vi "Cleanup.vi"(8 "error in (no error)":errorcluster, 11 "Shadow in":refnum<class "Shadow.lvclass">) -> (0 "error out":errorcluster)   [LabVIEW 2021, in "UIShadow.lvlib" / "Shadow.lvclass"]
uses:
  Shadow.lvclass
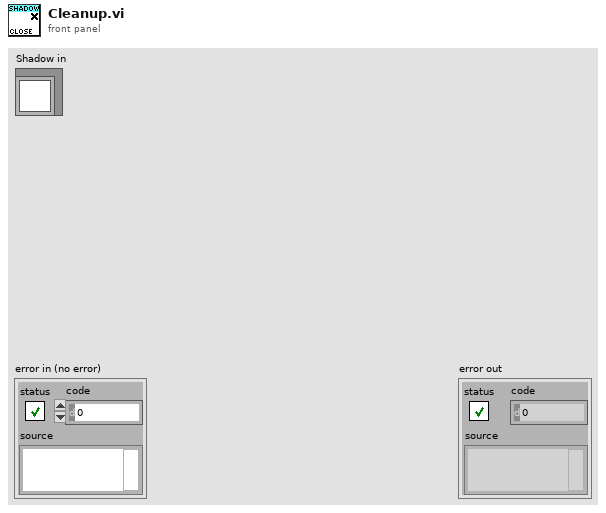
[diagram p1: front panel]
types:
  T1 = typedef "UIShadow.lvlib/Shadow.lvclass/Data.ctl" = cluster{"VI Refnum":refnum<vi>, "ShadowColor":u32, "Offset":i16, "Transparancy":i32, "UIShadowRef":refnum<vi>, "Activate?":bool}
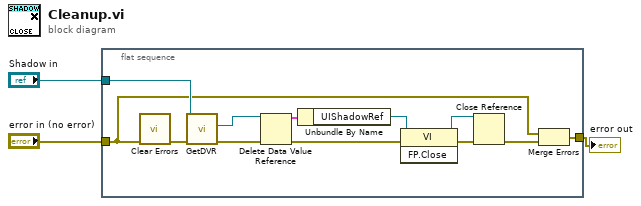
[diagram p0: block diagram]
diagram:
  n1 = flat-sequence {
    tunnel: "Shadow in" -> [w15]
    tunnel: [w13] -> w2
    tunnel: "error in (no error)" -> [w12]
    frame #0 {
      n2 = call <vilib>:"Clear Errors.vi"("error in (no error)"=w12) -> ("error out"=w14:errorcluster)  [unwired: 5 in, 1 out]
      n3 = call "GetDVR.vi"("error in (no error)"=w14, "Shadow in"=w15) -> ("error out"=w11:errorcluster, "DVR"=w9:refnum<data-value>)  [unwired: 7 in, 1 out]
      n4 = Delete Data Value Reference(data value reference=w9, error in=w11) -> (data value=w8:T1, error out=w10:errorcluster)
      n5 = Unbundle By Name(w8) -> ("UIShadowRef"=w5:refnum<vi>)
      n6 = invoke class="VI" method="FP.Close"(reference=w5, error in=w10) -> (reference out=w4:refnum<vi>, error out=w6:errorcluster)  [unwired: 1 in, 1 out]
      n7 = Close Reference(reference=w4, error in (no error)=w6) -> (error out=w7:errorcluster)
      n8 = Merge Errors(w12, w7) -> (w13:errorcluster)
    }
  }
  "error out" <- w2
